vi "semaphore_test.vi"   [LabVIEW 2013]
uses:
  Classes/Instrument/instrument.lvclass
panel:
  # "look at the wire diagram"
types:
  T1 = typedef "Semaphore RefNum" = refnum<k1>
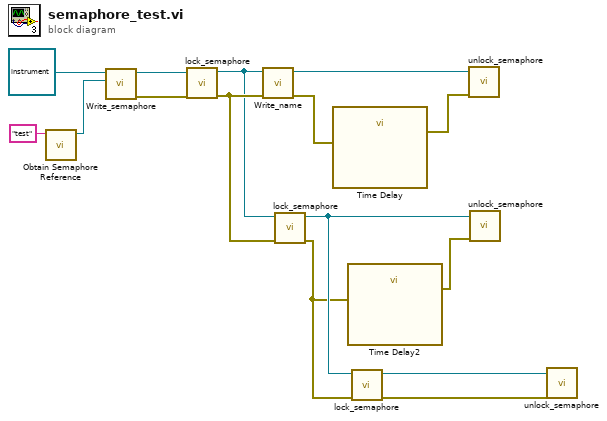
[diagram p0: block diagram]
diagram:
  n1 = call <vilib>:"Obtain Semaphore Reference.vi"("name (unnamed)"="test") -> ("semaphore"=w13:T1)  [unwired: 4 in, 2 out]
  n2 = call-dynamic "Write_semaphore.vi"("semaphore"=w13, "instrument in"=refnum<class "instrument.lvclass"> refnum ("instrument.lvclass")) -> ("error out"=w11:errorcluster, "instrument out"=w12:refnum<class "instrument.lvclass">)  [unwired: 8 in]
  n3 = call-dynamic "lock_semaphore.vi"("error in (no error)"=w11, "instrument in"=w12) -> ("error out"=w7:errorcluster, "instrument out"=w6:refnum<class "instrument.lvclass">)  [unwired: 8 in]
  n4 = call-dynamic "Write_name.vi"("error in (no error)"=w7, "instrument in"=w6) -> ("error out"=w10:errorcluster, "instrument out"=w8:refnum<class "instrument.lvclass">)  [unwired: 8 in]
  n5 = call-dynamic "lock_semaphore.vi"("error in (no error)"=w7, "instrument in"=w6) -> ("error out"=w2:errorcluster, "instrument out"=w3:refnum<class "instrument.lvclass">)  [unwired: 8 in]
  n6 = call "Time Delay"("error in (no error)"=w10) -> ("error out"=w9:errorcluster)  [unwired: 10 in]
  n7 = call "Time Delay2"("error in (no error)"=w2) -> ("error out"=w1:errorcluster)  [unwired: 10 in]
  n8 = call-dynamic "lock_semaphore.vi"("error in (no error)"=w2, "instrument in"=w3) -> ("error out"=w5:errorcluster, "instrument out"=w4:refnum<class "instrument.lvclass">)  [unwired: 8 in]
  n9 = call-dynamic "unlock_semaphore.vi"("error in (no error)"=w9, "instrument in"=w8) -> ()  [unwired: 8 in, 2 out]
  n10 = call-dynamic "unlock_semaphore.vi"("error in (no error)"=w1, "instrument in"=w3) -> ()  [unwired: 8 in, 2 out]
  n11 = call-dynamic "unlock_semaphore.vi"("error in (no error)"=w5, "instrument in"=w4) -> ()  [unwired: 8 in, 2 out]
